vi "4Pi AA Get Image.vi"(0 "Camera Notifier Name":string, 5 "Image Ref":T1, 7 "Frame Accums.":u16, 11 "Error In":errorcluster) -> (8 "Image Out":u16[][](array[numeric]), 15 "Error Out":errorcluster)   [LabVIEW 2020]
uses:
  <vilib>/vision/Image Controls.llb/IMAQ Image.ctl
  Device Library/Cameras/Hamamatsu/Orca Flash/Orca Flash Controls/Orca Flash Actions.ctl
  Display Module/Display Module Custom Controls/ROI Descriptor.ctl
  Device Library/Cameras/Camera Controls/Camera IMAQ Key Info.ctl
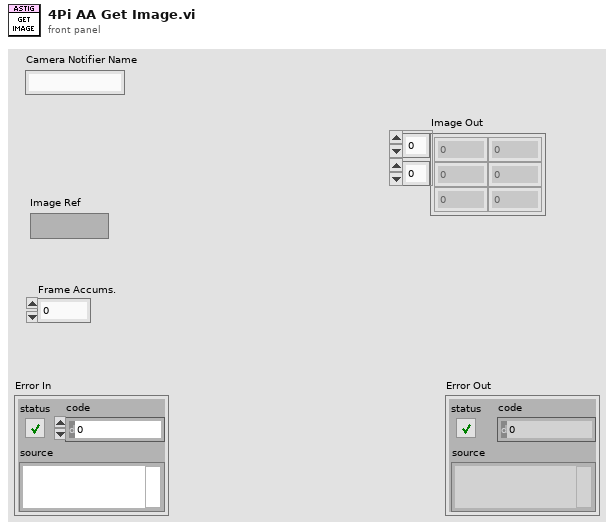
[diagram p1: front panel]
types:
  T1 = typedef "IMAQ Image.ctl" = refnum<image>
  T2 = typedef "ROI Descriptor.ctl" = cluster{"Global Rectangle":i32[], "Contours":cluster{"Contour Type":u32, "ROI Type":u32, "Points":i32[]}[]}
  T3 = typedef "Orca Flash Actions.ctl" = enum16{"IDLE", "PREVIEW", "RECORD", "Record Settings", "SETPARAM", "GETPARAM", "SETROI", "GETROI", "PROGRESSIVE MODE", "AREA MODE", "STATUS", "QUIT"}
  T4 = typedef "Camera IMAQ Key Info.ctl" = cluster{"Frame":u32, "Sensor Height":i32, "Sensor Width":i32, "ROI Height":i32, "ROI Width":i32, "ROI Enable?":bool, "Bit per Pixel":u8}
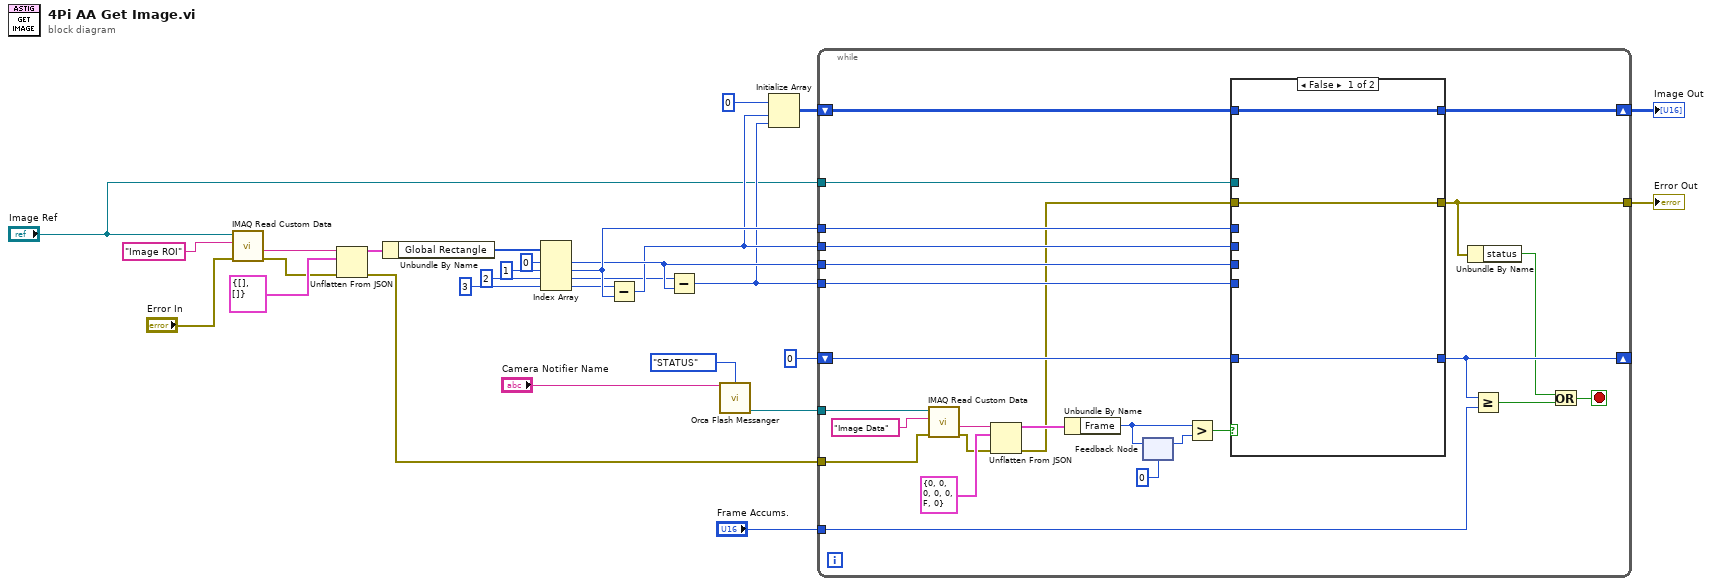
[diagram p0: block diagram]
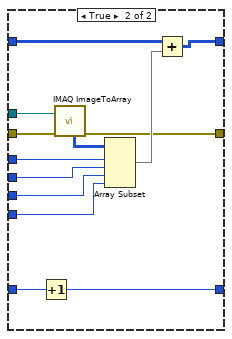
[diagram p2: hidden frame]
diagram:
  n1 = call "IMAQ Read Custom Data"("error in (no error)"="Error In", "Key"="Image ROI", "Image"="Image Ref") -> ("error out"=w3:errorcluster, "Custom Data Out"=w16:string)  [unwired: 6 in, 1 out]
  n2 = Unflatten From JSON(JSON string=w16, type and defaults=T2 {"Global Rectangle"=[], "Contours"=[]} ("Image ROI Descriptor"), error in (no error)=w3) -> (value=w14:T2, error out=w2:errorcluster)  [unwired: 4 in]
  n3 = Unbundle By Name(w14) -> ("Global Rectangle"=w13:i32[])
  n4 = Index Array(array=w13, index #1=0 ("index"), index #2=1 ("index"), index #3=2 ("index"), index #4=3 ("index")) -> (element #1=w21:i32, element #2=w22:i32, element #3=w7:i32, element #4=w8:i32)
  n5 = Subtract(x=w8, y=w22) -> (x-y=w20:i32)
  n6 = Subtract(x=w7, y=w21) -> (x-y=w19:i32)
  n7 = call "Orca Flash Messanger.vi"("Notifier Name"="Camera Notifier Name", "Camera Actions"=Orca_Flash_Actions."STATUS") -> ("Image Ref"=w26:T1)  [unwired: 9 in, 4 out]
  n8 = Initialize Array(u16 0, w20, w19) -> (w24:u16[][])
  n9 = while {
    tunnel: w26 -> [w50]
    shift-right: [w44] -> _
    shift-left: u16 0 -> [w45]
    tunnel: "Image Ref" -> [w43]
    shift-right: [w37] -> w18
    shift-left: w24 -> [w38]
    tunnel: w22 -> [w42]
    tunnel: w20 -> [w41]
    tunnel: w21 -> [w40]
    tunnel: w19 -> [w39]
    tunnel: "Frame Accums." -> [w36]
    tunnel: w2 -> [w35]
    tunnel: [w32] -> w1
    stop <- w29 stop-if-true
    n10 = call "IMAQ Read Custom Data"("error in (no error)"=w35, "Key"="Image Data", "Image"=w50) -> ("error out"=w34:errorcluster, "Custom Data Out"=w52:string)  [unwired: 6 in, 1 out]
    n11 = Unflatten From JSON(JSON string=w52, type and defaults=T4 {"Frame"=0, "Sensor Height"=0, "Sensor Width"=0, "ROI Height"=0, "ROI Width"=0, "ROI Enable?"=FALSE, "Bit per Pixel"=0} ("Camera IMAQ Key Info"), error in (no error)=w34) -> (value=w54:T4, error out=w33:errorcluster)  [unwired: 4 in]
    n12 = Unbundle By Name(w54) -> ("Frame"=w47:u32)
    n13 = feedback #1(u32 0 ("Frame")) -> (w49:u32)
    n14 = feedback-in #1(w47) -> ()
    n15 = Greater?(x=w47, y=w49) -> (0:w46:bool)
    n16 = case shown="False" w46 {
      tunnel: w45 -> [w57 w70]
      tunnel: [w57 w69] -> w44
      tunnel: w43 -> [_ w68]
      tunnel: w42 -> [_ w66]
      tunnel: w41 -> [_ w65]
      tunnel: w40 -> [_ w64]
      tunnel: w39 -> [_ w63]
      tunnel: w38 -> [w56 w62]
      tunnel: [w56 w60] -> w37
      tunnel: w33 -> [w55 w59]
      tunnel: [w55 w58] -> w32
      frame False {
      }
      frame True {
        n17 = Increment(x=w70) -> (x+1=w69:u16)
        n18 = call "IMAQ ImageToArray"("error in (no error)"=w59, "Image"=w68) -> ("Image Pixels (U16)"=w67:u16[][], "error out"=w58:errorcluster)  [unwired: 2 in, 3 out]
        n19 = Array Subset(array=w67, index (row)=w66, length (row)=w65, index (col)=w64, length (col)=w63) -> (w61:u16[][])
        n20 = Add(x=w62, y=w61) -> (x+y=w60:u16[][])
      }
    }
    n21 = Unbundle By Name(w32) -> ("status"=w30:bool)
    n22 = Greater Or Equal?(x=w44, y=w36) -> (x >= y?=w31:bool)
    n23 = Or(x=w30, y=w31) -> (x .or. y?=w29:bool)
  }
  "Image Out" <- w18
  "Error Out" <- w1
